vi "QX_DAQ Config.vi"(8 "error in":errorcluster, 10 "InUsedDevRef[]":T3(array[cluster]), 11 "InUsedChan[]":T2) -> (0 "error out":errorcluster caption="Error out", 3 "DaqMeasurement":refnum<k24>)   [LabVIEW 2016]
uses:
  Ctrls/HardWare _ Channel Parameters.ctl
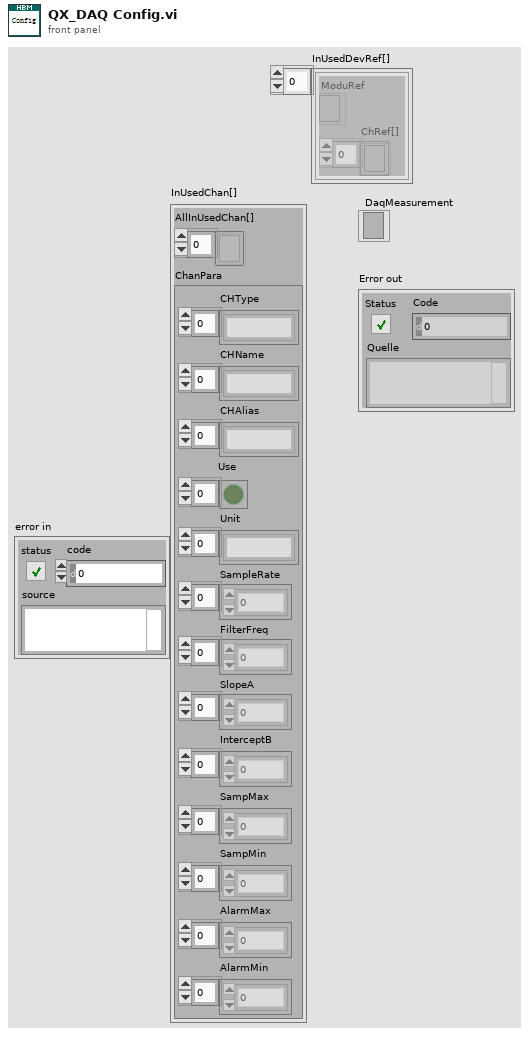
[diagram p1: front panel]
types:
  T1 = typedef "HardWare _ Channel Parameters.ctl" = cluster{"CHType":string[], "CHName":string[], "CHAlias":string[], "Use":bool[], "Unit":string[], "SampleRate":dbl[], "FilterFreq":dbl[], "SlopeA":dbl[], "InterceptB":dbl[], "SampMax":dbl[], "SampMin":dbl[], "AlarmMax":dbl[], "AlarmMin":dbl[]}
  T2 = cluster{"AllInUsedChan[]":refnum<k24>[], "ChanPara":T1}
  T3 = cluster{"ModuRef":refnum<k24>, "ChRef[]":refnum<k24>[]}[]
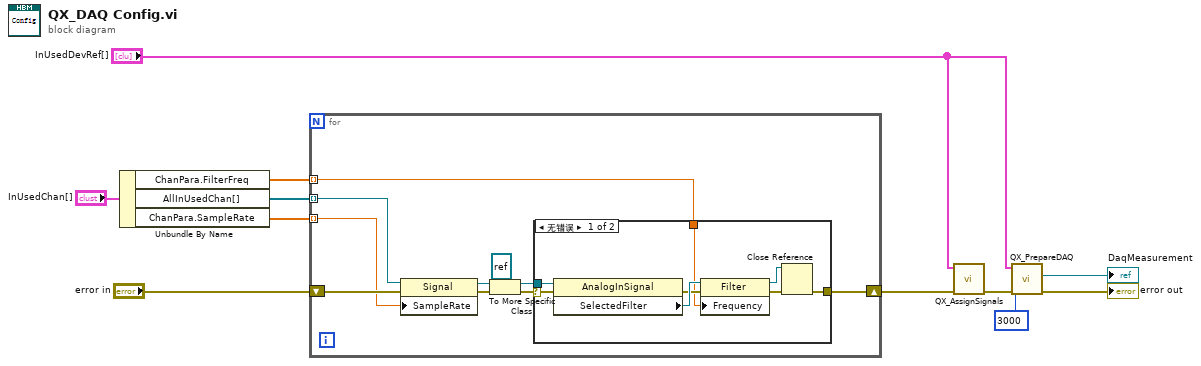
[diagram p0: block diagram]
diagram:
  n1 = Unbundle By Name("InUsedChan[]") -> ("ChanPara.FilterFreq"=w3:dbl[], "AllInUsedChan[]"=w1:refnum<k24>[], "ChanPara.SampleRate"=w2:dbl[])
  n2 = for {
    shift-right: [w20] -> w10
    shift-left: "error in" -> [w21]
    tunnel: w3 -> [w14] mode=indexing
    tunnel: w2 -> [w13] mode=indexing
    tunnel: w1 -> [w12] mode=indexing
    n3 = property on="Eigenschaftsknoten" class="Signal"(reference=w12, error in=w21, "SampleRate"=w13) -> (reference out=w15:refnum<k24>, error out=w18:errorcluster)
    n4 = To More Specific Class(target class=refnum<k24> refnum (".NET (Referenz)"), reference=w15, error in=w18) -> (specific class reference=w17:refnum<k24>, error out=w16:errorcluster)
    n5 = case shown="无错误" w16 {
      selector: w16 -> [w27 w30]
      tunnel: w17 -> [w29 _]
      tunnel: [w23 w30] -> w20
      tunnel: w14 -> [w22 _]
      frame No Error {
        n6 = property on="Eigenschaftsknoten" class="AnalogInSignal"(reference=w29, error in=w27) -> (error out=w26:errorcluster, "SelectedFilter"=w28:refnum<k24>)  [unwired: 1 out]
        n7 = property on="Eigenschaftsknoten" class="Filter"(reference=w28, error in=w26, "Frequency"=w22) -> (reference out=w24:refnum<k24>, error out=w25:errorcluster)
        n8 = Close Reference(reference=w24, error in (no error)=w25) -> (error out=w23:errorcluster)
      }
      frame Error {
      }
    }
  }
  n9 = call "QX_AssignSignals.vi"("Error in"=w10, "DevRef[]"="InUsedDevRef[]") -> ("Error out"=w9:errorcluster)  [unwired: 9 in]
  n10 = call "QX_PrepareDAQ.vi"("Error in"=w9, "BufferTimeout"=3000, "DevRef[]"="InUsedDevRef[]") -> ("Error out"=→"error out":errorcluster, "DaqMeasurement"=→"DaqMeasurement":refnum<k24>)  [unwired: 7 in]
